vi "SNMP Parse Sequence Data.vi"(1 "Sequence Data":u8[](array[numeric]) format="%.0x") -> (0 "SequenceAsStrings":string[][](array[string]))   [LabVIEW 2017]
doc: "This VI ise used to parse the variable bindings list of a SNMP PDU. The data is input as a byte arrays and the output is a 2D array of strings. Each row of the output array represents an ASCII representation of the OID, type, and value contained in the variable binding list."
uses:
  CTL - SNMP Types.ctl
panel:
  in  "SNMP Data Types":T1={"Integer"=2, "Octet-String"=4, "NULL"=5, "Object Identifier"=6, "Sequence"=48, "IP Address"=64, "Counter"=65, "Gauge"=66, "TimeTicks"=67, "Opaque"=68, "GetRequest-PDU"=160, "GetNextRequest-PDU"=161, "GetResponse-PDU"=162, "SetRequest-PDU"=163, "Trap-PDU"=164} {"Opaque" format="%.0x"; "TimeTicks" format="%.0x"; "Gauge" format="%.0x"; "Counter" format="%.0x"; "IP Address" format="%.0x"; "NULL" format="%.0x"; "Trap-PDU" format="%.0x"; "SetRequest-PDU" format="%.0x"; "GetNextRequest-PDU" format="%.0x"; "Object Identifier" format="%.0x"; "Sequence" format="%.0x"; "GetResponse-PDU" format="%.0x"; "GetRequest-PDU" format="%.0x"; "Octet-String" format="%.0x"; "Integer" format="%.0x"}
  out "SeqDataArray":u8[][](array[numeric]) format="%.0x"
  out "Sequence Length":u8
  out "Varbind-index":u8[](array[numeric]) format="%.0x"
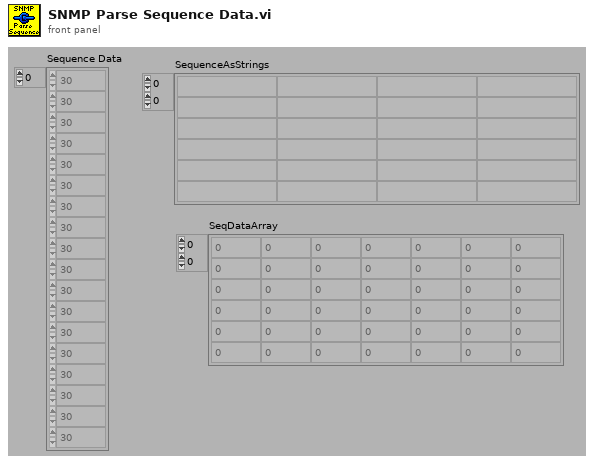
[diagram p1: front panel]
types:
  T1 = typedef "CTL - SNMP Types.ctl" = cluster{"Integer":u8, "Octet-String":u8, "NULL":u8, "Object Identifier":u8, "Sequence":u8, "IP Address":u8, "Counter":u8, "Gauge":u8, "TimeTicks":u8, "Opaque":u8, "GetRequest-PDU":u8, "GetNextRequest-PDU":u8, "GetResponse-PDU":u8, "SetRequest-PDU":u8, "Trap-PDU":u8}
  T2 = cluster{"Numeric":u32, "Octet String":string, "Byte Array":u8[]}
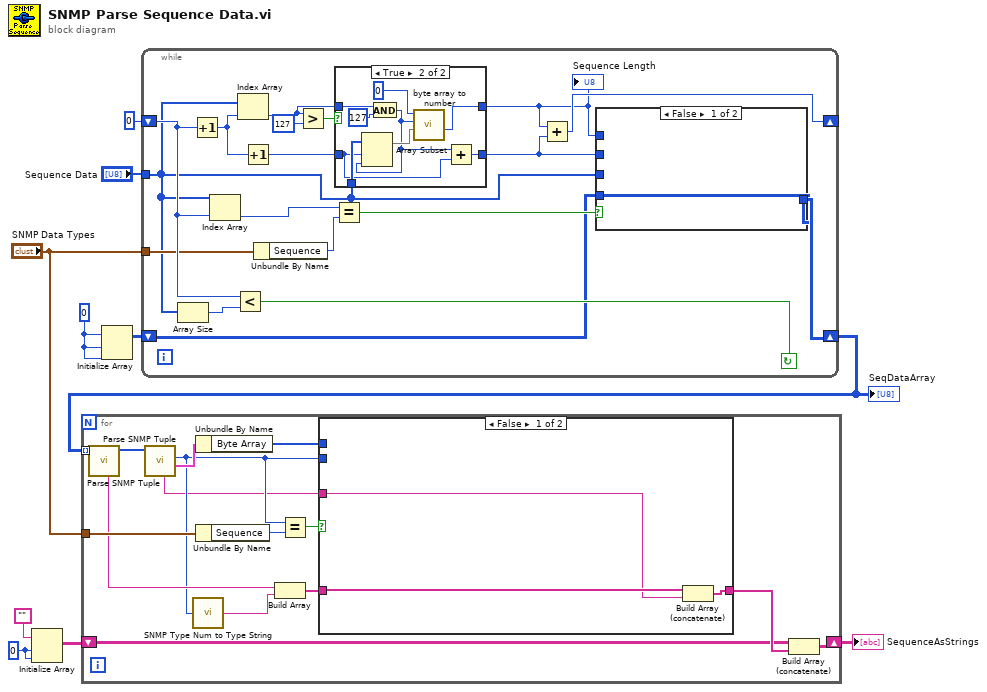
[diagram p0: block diagram]
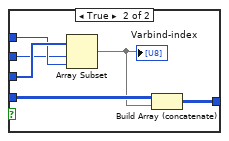
[diagram p3: hidden frame]
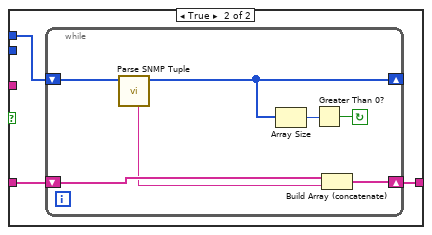
[diagram p4: hidden frame]
diagram:
  w4 = 0
  w6 = u8 0
  n1 = Initialize Array("", w4, w4) -> (w3:string[][])
  n2 = Initialize Array(w6, w6, w6) -> (w7:u8[][])
  n3 = while {
    tunnel: "SNMP Data Types" -> [w19]
    shift-left: w7 -> [w21]
    shift-right: [w20] -> w8
    shift-left: 0 -> [w23]
    shift-right: [w22] -> _
    tunnel: "Sequence Data" -> [w11]
    stop <- w24 continue-if-true
    n4 = Array Size(array=w11) -> (size(s)=w25:i32)
    n5 = Increment(x=w23) -> (x+1=w13:u32)
    n6 = Index Array(array=w11, index=w23) -> (element=w28:u8)
    n7 = Less?(x=w23, y=w25) -> (x < y?=w24:bool)
    n8 = Index Array(array=w11, index=w13) -> (element=w16:u8)
    n9 = Increment(x=w13) -> (x+1=w12:u32)
    n10 = Unbundle By Name(w19) -> ("Sequence"=w27:u8)
    n11 = Greater?(x=w16, y=u8 127) -> (0:w17:bool)
    n12 = Equal?(x=w28, y=w27) -> (x = y?=w26:bool)
    n13 = case shown="True" w17 {
      tunnel: w16 -> [w30 w38]
      tunnel: w12 -> [w29 w32]
      tunnel: [w30 w34] -> w15
      tunnel: [w29 w31] -> w14
      tunnel: w11 -> [_ w39]
      frame False {
      }
      frame True {
        n14 = And(x=w38, y=u8 127) -> (x .and. y?=w33:u8)
        n15 = Array Subset(array=w39, index=w32, length=w33) -> (w36:u8[])
        n16 = call "byte array to number.vi"("Byte Array"=w36, "Byte Length"=w33, "Start Value"=u32 0) -> ("Number"=w34:u32)  [unwired: 8 out]
        n17 = Add(x=w33, y=w32) -> (x+y=w31:u32)
      }
    }
    "Sequence Length" <- w15
    n18 = Add(x=w15, y=w14) -> (x+y=w22:u32)
    n19 = case shown="False" w26 {
      tunnel: w11 -> [_ w46]
      tunnel: w15 -> [_ w45]
      tunnel: w14 -> [_ w44]
      tunnel: w21 -> [w40 w43]
      tunnel: [w40 w41] -> w20
      frame False {
      }
      frame True {
        n20 = Array Subset(array=w46, index=w44, length=w45) -> (w42:u8[])
        "Varbind-index" <- w42
        n21 = Build Array (concatenate)(w43, w42) -> (w41:u8[][])
      }
    }
  }
  "SeqDataArray" <- w8
  n22 = for {
    tunnel: w8 -> [w56] mode=indexing
    shift-right: [w58] -> w2
    shift-left: w3 -> [w57]
    tunnel: "SNMP Data Types" -> [w60]
    n23 = call "Parse SNMP Tuple.vi"("SNMP Packet In"=w56) -> ("SNMP Packet Out"=w48:u8[], "Data As String"=w55:string)  [unwired: 1 in, 8 out]
    n24 = call "Parse SNMP Tuple.vi"("SNMP Packet In"=w48) -> ("Data Out"=w61:T2, "Data Type"=w50:u8, "Data As String"=w49:string)  [unwired: 1 in, 7 out]
    n25 = call "SNMP Type Num to Type String.vi"("Type"=w50) -> ("StringForType"=w51:string)
    n26 = Unbundle By Name(w61) -> ("Byte Array"=w47:u8[])
    n27 = Unbundle By Name(w60) -> ("Sequence"=w52:u8)
    n28 = Build Array(w55, w51) -> (w54:string[])
    n29 = Equal?(x=w50, y=w52) -> (x = y?=w53:bool)
    n30 = case shown="False" w53 {
      tunnel: [w63 w67] -> w59
      tunnel: w47 -> [_ w65]
      tunnel: w54 -> [w64 w66]
      tunnel: w50 -> [_ _]
      tunnel: w49 -> [w62 _]
      frame False {
        n31 = Build Array (concatenate)(w64, w62) -> (w63:string[])
      }
      frame True {
        n32 = while {
          shift-left: w66 -> [w73]
          shift-right: [w71] -> w67
          shift-left: w65 -> [w74]
          shift-right: [w70] -> _
          stop <- w68 continue-if-true
          n33 = call "Parse SNMP Tuple.vi"("SNMP Packet In"=w74) -> ("SNMP Packet Out"=w70:u8[], "Data As String"=w72:string)  [unwired: 1 in, 8 out]
          n34 = Array Size(array=w70) -> (size(s)=w69:i32)
          n35 = Greater Than 0?(x=w69) -> (x > 0?=w68:bool)
          n36 = Build Array (concatenate)(w73, w72) -> (w71:string[])
        }
      }
    }
    n37 = Build Array (concatenate)(w57, w59) -> (w58:string[][])
  }
  "SequenceAsStrings" <- w2
